vi "Auton_Selector.vi"(11 "Auton Name In":string) -> (3 "Auton Steps":T1[](array[typedef]))   [LabVIEW 2019]
uses:
  Auton Subsystems Steps Typedef.ctl
  Drive/Drive Command Typedef.ctl
  Drive/Drive Mode Typedef.ctl
  Shoot/Shooter Command Type Def.ctl
  Shoot/Shooter Mode Type Def.ctl
  Shoot/Shooter Preset speeds Type Def.ctl
  Intake/Intake Command Type Def.ctl
  Intake/Intake Mode Type Def.ctl
  <vilib>/Rock Robotics/WPI/Solenoid/WPI_SolenoidValue.ctl
panel:
  in  "Possible autons":T10(array[cluster])
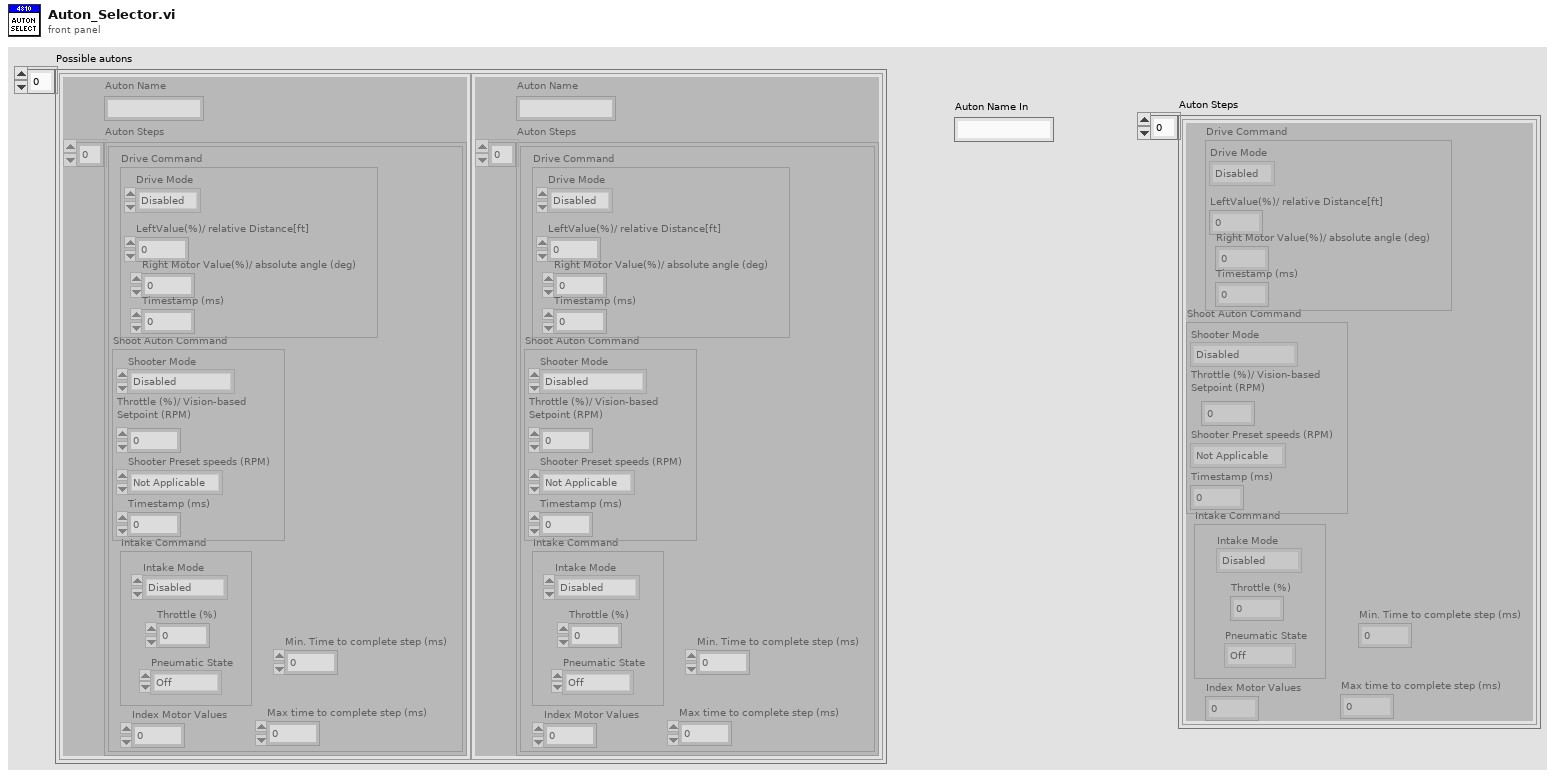
[diagram p1: front panel]
types:
  T1 = typedef "Auton Subsystems Steps Typedef.ctl" = cluster{"Drive Command":T2, "Shoot Auton Command":T4, "Intake Command":T7, "Index Motor Values":dbl, "Max time to complete step (ms)":dbl, "Min. Time to complete step (ms)":dbl}
  T2 = typedef "Drive Command Typedef.ctl" = cluster{"Drive Mode":T3, "LeftValue(%)/ relative Distance[ft]":dbl, "Right Motor Value(%)/ absolute angle (deg)":dbl, "Timestamp (ms)":dbl}
  T3 = typedef "Drive Mode Typedef.ctl" = enum16{"Disabled", "Auto-align", "Drive Distance", "Turn to angle", "Driver"}
  T4 = typedef "Shooter Command Type Def.ctl" = cluster{"Shooter Mode":T5, "Throttle (%)/ Vision-based\nSetpoint (RPM)":dbl, "Shooter Preset speeds (RPM)":T6, "Timestamp (ms)":dbl}
  T5 = typedef "Shooter Mode Type Def.ctl" = enum16{"Disabled", "Raw Throttle", "Preset Velocity Control", "Vision-based Velocity Control"}
  T6 = typedef "Shooter Preset speeds Type Def.ctl" = enum16{"Not Applicable", "Target Zone", "Initiation Line", "Close end of Trench Run", "Control Panel"}
  T7 = typedef "Intake Command Type Def.ctl" = cluster{"Intake Mode":T8, "Throttle (%)":dbl, "Pneumatic State":T9}
  T8 = typedef "Intake Mode Type Def.ctl" = enum16{"Disabled", "Enabled"}
  T9 = typedef "WPI_SolenoidValue.ctl" = enum16{"Off", "On", "Forward", "Reverse"}
  T10 = cluster{"Auton Name":string, "Auton Steps":T1[]}[]
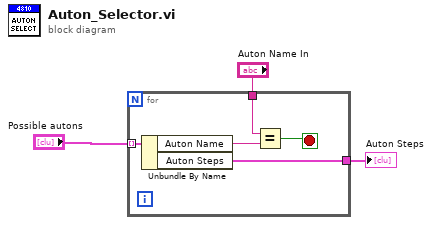
[diagram p0: block diagram]
diagram:
  n1 = for {
    tunnel: "Possible autons" -> [w8] mode=indexing
    tunnel: "Auton Name In" -> [w6]
    tunnel: [w4] -> w1
    stop <- w5 stop-if-true
    n2 = Unbundle By Name(w8) -> ("Auton Name"=w7:string, "Auton Steps"=w4:T1[])
    n3 = Equal?(x=w6, y=w7) -> (x = y?=w5:bool)
  }
  "Auton Steps" <- w1
